vi "MyG#G3SubTempl_SetModifiedClassAttributes.vi"(0 "reference in":refnum<class "MyG#G3SubTempl.lvclass">, 2 "attributes":T1, 3 "Only unlock data? (F)":bool, 4 "Unlock data if error? (T)":bool=TRUE, 5 "error in (no error)":errorcluster, 7 "Update data even if error? (F)":bool) -> (14 "reference out":refnum<class "MyG#G3SubTempl.lvclass">, 19 "error out":errorcluster)   [LabVIEW 2020, in "MyG#G3SubTempl.lvclass"]
doc: "This VI overwrites the attributes associated with the object reference and unlocks it for write access. If error in is set, the object is unlocked but its data will not be modified.\n\nIn order to use this VI, you must first successfully lock the object's data using this class GetAttributesToModify VI."
uses:
  MyG#G3SubTempl.lvclass
  C:/Program Files (x86)/National Instruments/LabVIEW 2020/examples/AddQ/G#/CreateDestroy/MyG#G3Templ_class/MyG#G3Templ.lvclass
  protected/ClassAttributes.ctl
  MyG#G3Templ_class/protected/ClassAttributes.ctl
  MyG#G3SubTempl.lvclass/MyG#G3SubTempl.ctl
  MyG#G3Templ_class/MyG#G3Templ.lvclass
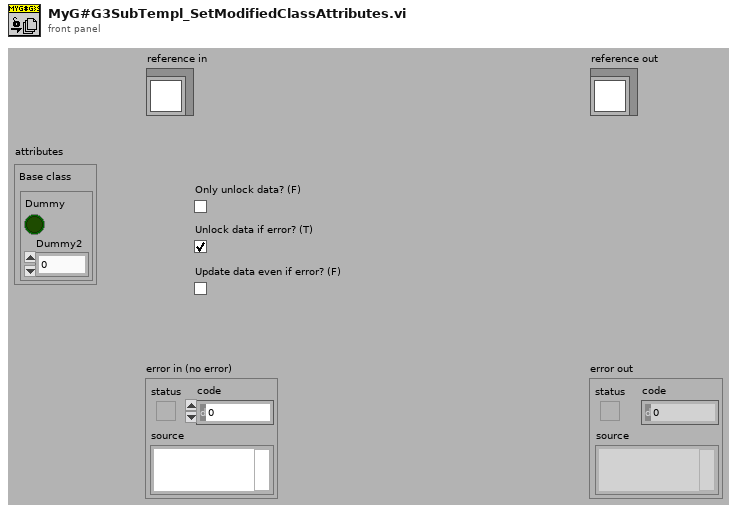
[diagram p1: front panel]
types:
  T1 = typedef "MyG#G3SubTempl.lvclass/ClassAttributes.ctl" = cluster{"Base class":T2}
  T2 = typedef "MyG#G3Templ.lvclass/ClassAttributes.ctl" = cluster{"Dummy":bool, "Dummy2":dbl}
  T3 = typedef "MyG#G3SubTempl.lvclass/ClassAttributesRef.ctl" = refnum<data-value>
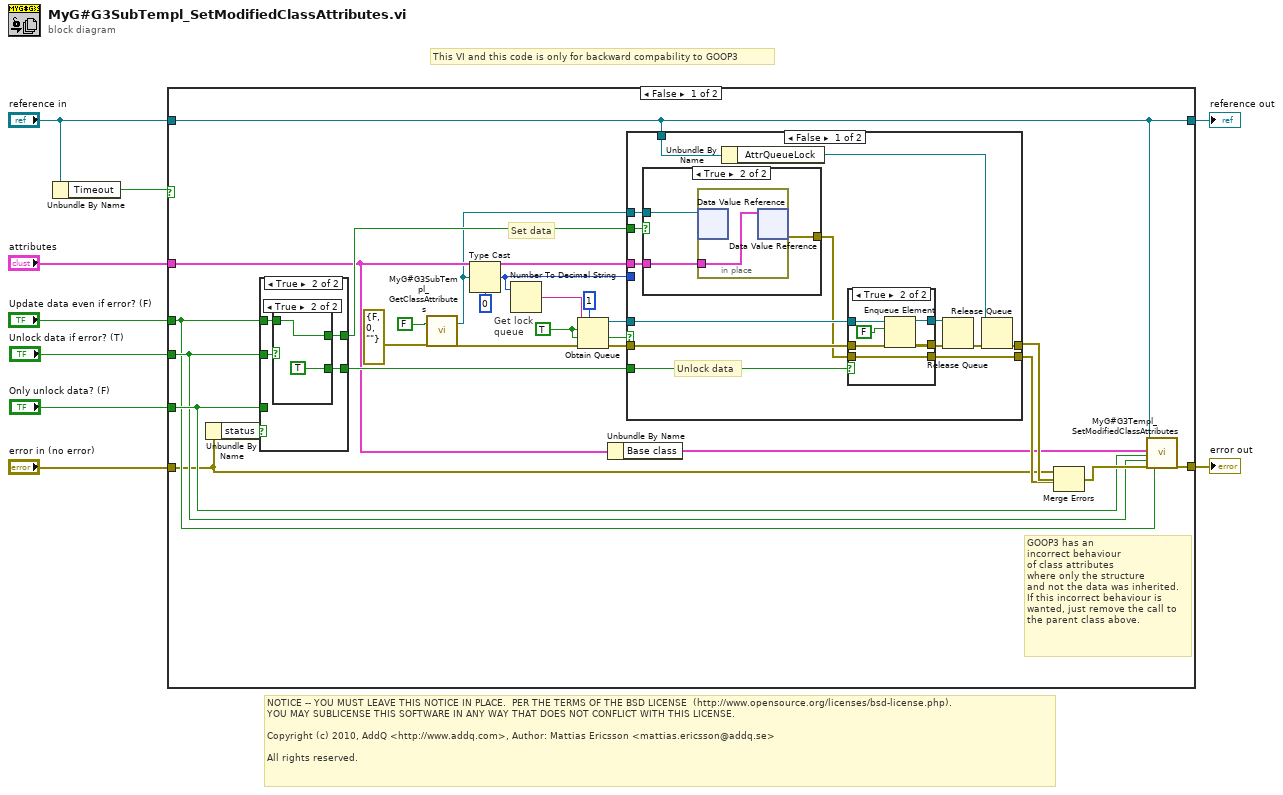
[diagram p0: block diagram]
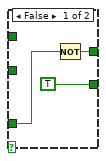
[diagram p2: hidden frame]
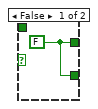
[diagram p3: hidden frame]
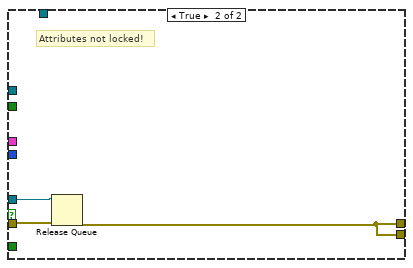
[diagram p6: hidden frame]
diagram:
  # "NOTICE -- YOU MUST LEAVE THIS NOTICE IN PLACE.  PER THE TERMS OF THE BSD LICENSE  (http://www.opensource.org/licenses/bsd-license.php).\nYOU MAY SUBLICENSE THIS SOFTWARE IN ANY WAY THAT DOES NOT CONFLICT WITH THIS LICENSE.\n\nCopyright (c) 2010, AddQ <http://www.addq.com>, Author: Mattias Ericsson <mattias.ericsson@addq.se>\n\nAll rights reserved."
  # "This VI and this code is only for backward compability to GOOP3"
  n1 = Unbundle By Name("reference in") -> ("Timeout"=w1:bool)
  n2 = case shown="False" w1 {
    tunnel: [w21 w76] -> w9
    tunnel: "reference in" -> [w20 w77]
    tunnel: "error in (no error)" -> [w12 w76]
    tunnel: "attributes" -> [w19 _]
    tunnel: "Only unlock data? (F)" -> [w17 _]
    tunnel: "Unlock data if error? (T)" -> [w16 _]
    tunnel: "Update data even if error? (F)" -> [w15 _]
    tunnel: [w20 w77] -> w2
    frame False {
      w34 = TRUE ("create if not found? (T)")
      # "GOOP3 has an\nincorrect behaviour\nof class attributes\nwhere only the structure\nand not the data was inherited.\nIf this incorrect behaviour is\nwanted, just remove the call to\nthe parent class above."
      # "Get lock\nqueue"
      # "Set data"
      n3 = Unbundle By Name(w12) -> ("status"=w28:bool)
      n4 = case shown="True" w28 {
        tunnel: [w36 w41] -> w27
        tunnel: w17 -> [w38 _]
        tunnel: [TRUE w40] -> w26
        tunnel: w16 -> [_ w42]
        tunnel: w15 -> [_ w39]
        frame False {
          n5 = Not(x=w38) -> (.not. x?=w36:bool)
        }
        frame True {
          n6 = case shown="True" w42 {
            tunnel: [w43 w44] -> w41
            tunnel: [w43 TRUE] -> w40
            tunnel: w39 -> [_ w44]
            frame False {
              w43 = FALSE
            }
            frame True {
            }
          }
        }
      }
      n7 = call "MyG#G3SubTempl_GetClassAttributes.vi"("return data"=FALSE, "error in (no error)"=errorcluster {"status"=FALSE, "code"=0, "source"=""}) -> ("class attributes ref"=w13:T3, "error out"=w11:errorcluster)  [unwired: 13 in, 3 out]
      n8 = Type Cast(type=u32 0, x=w13) -> (*(type *) &x=w24:u32)
      n9 = Number To Decimal String(number=w24) -> (decimal integer string=w35:string)  [unwired: 1 in]
      n10 = Obtain Queue(max queue size (-1, unlimited)=1, name (unnamed)=w35, element data type=w34, create if not found? (T)=w34, error in (no error)=w11) -> (queue out=w30:refnum<queue>, created new?=w31:bool, error out=w32:errorcluster)
      n11 = Unbundle By Name(w19) -> ("Base class"=w18:T2)
      n12 = case shown="False" w31 {
        tunnel: w32 -> [w59 w74]
        tunnel: w30 -> [w58 w73]
        tunnel: [w52 w75] -> w29
        tunnel: w24 -> [_ _]
        tunnel: w27 -> [w55 _]
        tunnel: w19 -> [w54 _]
        tunnel: w26 -> [w53 _]
        tunnel: w20 -> [w50 _]
        tunnel: [w47 w75] -> w23
        tunnel: w13 -> [w46 _]
        frame False {
          # "Unlock data"
          n13 = case shown="True" w55 {
            tunnel: w54 -> [_ w71]
            tunnel: [_ w70] -> w48
            tunnel: w46 -> [_ w69]
            frame False {
            }
            frame True {
              n14 = in-place {
                in-place-border: w71 -> [w72]
                n15 = in-place-dvr #1(w69) -> ()  [unwired: 2 out]
                n16 = in-place-dvr #1(w72) -> (w70:errorcluster)  [unwired: 1 out]
              }
            }
          }
          n17 = Unbundle By Name(w50) -> ("AttrQueueLock"=w49:refnum<queue>)
          n18 = case shown="True" w53 {
            tunnel: w59 -> [w61 w68]
            tunnel: w58 -> [w62 w67]
            tunnel: [w61 w66] -> w57
            tunnel: [w62 w65] -> w56
            tunnel: w48 -> [w60 w63]
            tunnel: [w60 w63] -> w47
            frame False {
            }
            frame True {
              n19 = Enqueue Element(queue=w67, element=FALSE, error in (no error)=w68) -> (queue out=w65:refnum<queue>, error out=w66:errorcluster)  [unwired: 1 in, 1 out]
            }
          }
          n20 = Release Queue(queue=w56, error in (no error)=w57) -> (error out=w51:errorcluster)  [unwired: 1 in, 2 out]
          n21 = Release Queue(queue=w49, error in (no error)=w51) -> (error out=w52:errorcluster)  [unwired: 1 in, 2 out]
        }
        frame True {
          # "Attributes not locked!"
          n22 = Release Queue(queue=w73, error in (no error)=w74) -> (error out=w75:errorcluster)  [unwired: 1 in, 2 out]
        }
      }
      n23 = Merge Errors(w12, w29, w23) -> (w22:errorcluster)
      n24 = call "MyG#G3Templ_SetModifiedClassAttributes.vi"("reference in"=w20, "attributes"=w18, "Only unlock data? (F)"=w17, "Unlock data if error? (T)"=w16, "error in (no error)"=w22, "Update data even if error? (F)"=w15) -> ("error out"=w21:errorcluster)  [unwired: 12 in, 1 out]
    }
    frame True {
      # "Timeout or not locked!"
    }
  }
  "error out" <- w9
  "reference out" <- w2
